vi "串口自动测试结论.vi"(9 "232 or 485":i32, 11 "第几路":i32) -> ()   [LabVIEW 2010]
uses:
  全局量/自动测试结果.vi
panel:
  # "从1开始"
  # "0：RS232    1：RS485"
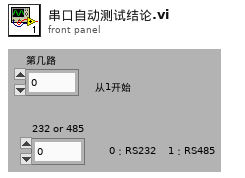
[diagram p1: front panel]
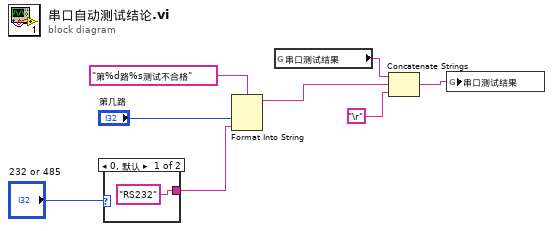
[diagram p0: block diagram]
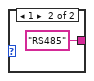
[diagram p2: hidden frame]
diagram:
  n1 = case shown="0, 默认" "232 or 485" {
    tunnel: ["RS232" "RS485"] -> w2
    frame 0, Default {
    }
    frame 1 {
    }
  }
  n2 = Format Into String(format string="第%d路%s测试不合格", "第几路", w2) -> (resulting string=w1:string)  [unwired: 2 in, 1 out]
  n3 = global read "自动测试结果.vi" "串口测试结果"() -> (w6:string)
  n4 = Concatenate Strings(w6, w1, "\r") -> (w8:string)
  n5 = global write "自动测试结果.vi" "串口测试结果"(w8) -> ()
